vi "Get Slider Min Max.vi"(11 "Slider":cluster{dbl, dbl}) -> (2 "min(x,y)":dbl, 3 "max(x,y)":dbl)   [LabVIEW 2015]
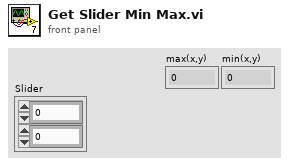
[diagram p1: front panel]
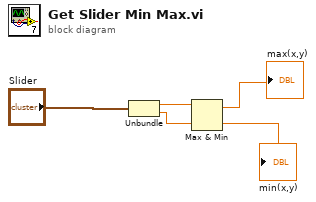
[diagram p0: block diagram]
diagram:
  n1 = Unbundle("Slider") -> (w2:dbl, w1:dbl)
  n2 = Max & Min(x=w2, y=w1) -> (max(x,y)=→"max(x,y)":dbl, min(x,y)=→"min(x,y)":dbl)
